vi "Get Drivers List.vi"(11 "error in (no error)":errorcluster) -> (4 "Drivers List Out":string[](array[string]), 6 "Total Driver List":i32, 8 "Removed Duplicates":string[](array[string]), 10 "Removed Duplicates Size":i32, 14 "Total Size":i32, 15 "error out":errorcluster)   [LabVIEW 2021, in "Converter Reusables.lvlib"]
uses:
  Converter Reusables.lvlib
  controls/Dictionary States.ctl
  77a78234-7449-441e-9ac3-41e4d218bce4.vi
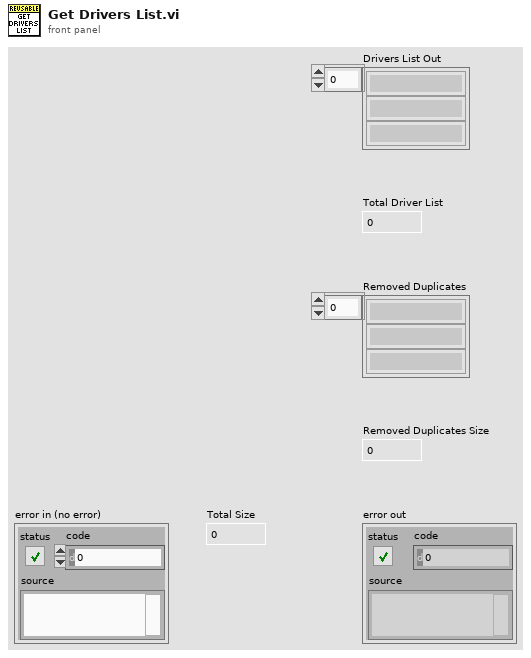
[diagram p1: front panel]
types:
  T1 = typedef "Converter Reusables.lvlib/Dictionary States.ctl" = enum16{"Set", "Get", "Delete", "Delete All"}
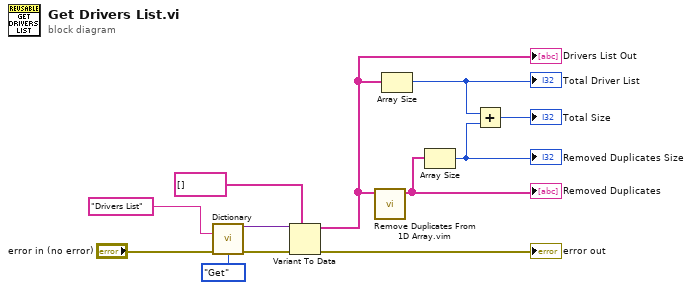
[diagram p0: block diagram]
diagram:
  n1 = call "Dictionary.vi"("Key"="Drivers List", "error in (no error)"="error in (no error)", "Dict States"=Dictionary_States."Get") -> ("Variant_Out"=w8:variant, "error out"=w9:errorcluster)  [unwired: 11 in]
  n2 = Variant To Data(error in=w9, type=string[] [], Variant=w8) -> (data=w5:string[], error out=→"error out":errorcluster)
  "Drivers List Out" <- w5
  n3 = call "Remove Duplicates From 1D Array.vim"("array"=w5) -> ("array with duplicates removed"=w4:string[])  [unwired: 10 in]
  "Removed Duplicates" <- w4
  n4 = Array Size(array=w5) -> (size(s)=w3:i32)
  "Total Driver List" <- w3
  n5 = Array Size(array=w4) -> (size(s)=w2:i32)
  "Removed Duplicates Size" <- w2
  n6 = Add(x=w3, y=w2) -> (x+y=→"Total Size":i32)
